vi "swiftCreate.vi"() -> ()   [LabVIEW 2016, in "Cerebellum.lvclass"]
uses:
  Cerebellum.lvclass
  Controls/Type of Synapses.ctl
  Cube/Grid.lvclass
  Cube/Grid.lvclass/Grid.ctl
  AER/AER.lvclass/AER.ctl
  Controls/Type of Neuron.ctl
  <vilib>/Utility/xml.llb/Write to XML File(string).vi
  <vilib>/Utility/file.llb/Write Delimited Spreadsheet.vi
  <vilib>/Utility/file.llb/Write Delimited Spreadsheet (DBL).vi
  <vilib>/Utility/xml.llb/Read From XML File(string).vi
  Synapses/Synapses.lvclass
  AER/AER.lvclass
panel:
  out "Creating grid":dbl(slide) scale=0.0..1.0
  in  "Show":bool
  in  "stop":bool
  in  "Create":bool
  out "Grid":string
  in  "Synapses and parameters":T2(array[cluster])=[{"Conv %"=4.0, "Synapse"=enum."MF to GC", "Weight Gain"=0.4}, {"Conv %"=4.0, "Synapse"=enum."GO to GC", "Weight Gain"=-0.03}, {"Conv %"=0.4, "Synapse"=enum."GC to GO", "Weight Gain"=0.002}, {"Conv %"=0.5, "Synapse"=enum."MF to GO", "Weight Gain"=0.001}, {"Conv %"=0.5, "Synapse"=enum."GC to PC", "Weight Gain"=0.003}, {"Conv %"=0.1, "Synapse"=enum."GC to BA", "Weight Gain"=0.008}, {"Conv %"=0.01, "Synapse"=enum."PC to BA", "Weight Gain"=-0.2}, {"Conv %"=0.4, "Synapse"=enum."BA to PC", "Weight Gain"=-0.01}, {"Conv %"=0.1, "Synapse"=enum."BA to GO", "Weight Gain"=-0.01}]
  in  "Prefix for output files name?":string="aer_"
  in  "How namy maps?":i32=1
  out "Preview":string
  in  "New":bool
  in  "Load":bool
  in  "Existing Grids in Results/":i32(listbox)
  # "Given the Grid, create random synaptic weights, distance based synaptic connections and output AER maps"
  # "Double click on the grid name shows details"
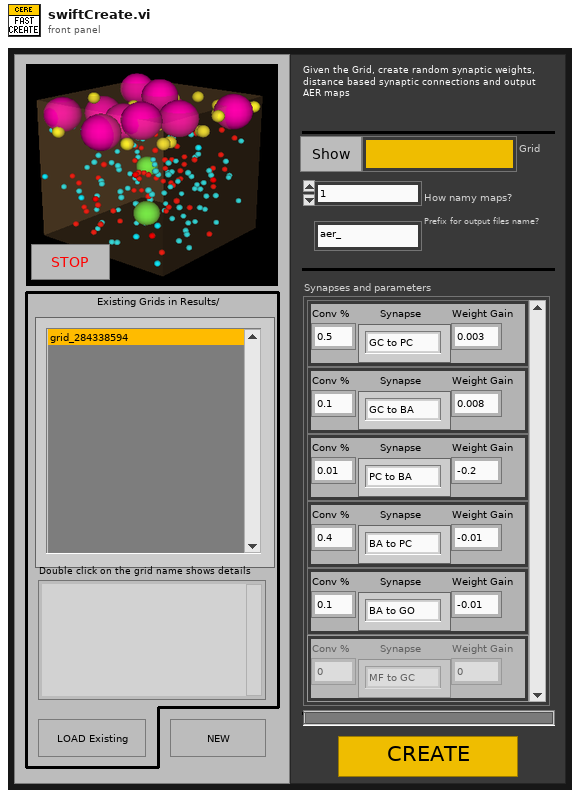
[diagram p1: front panel]
types:
  T1 = typedef "Type of Synapses.ctl" = enum16{"MF to GC", "GO to GC", "GC to GO", "MF to GO", "GC to PC", "GC to BA", "PC to BA", "BA to PC", "BA to GO"}
  T2 = cluster{"Conv %":dbl, "Synapse":T1, "Weight Gain":dbl}[]
  T3 = enum16{"Iddle", "CreateGrid", "CreateMaps", "LoadGrids", "Init", "ShowGrid"}
  T4 = enum8{"Enabled", "Disabled", "Disabled and Grayed Out"}
  T5 = enum16{"Iddle", "CreateGrid", "CreateMaps", "LoadGrids", "Init"}
  T6 = typedef "Type of Neuron.ctl" = enum16{"MF", "BA", "GO", "GC", "PC", "LU", "Glia (Dummy)"}
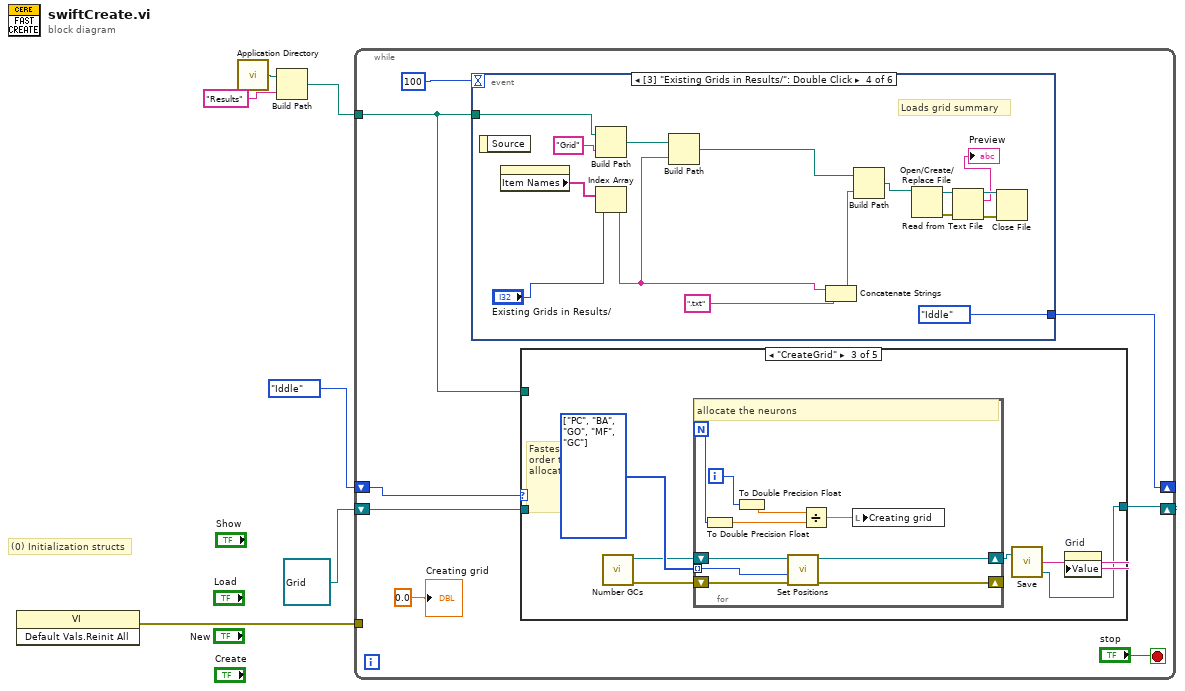
[diagram p0: block diagram]
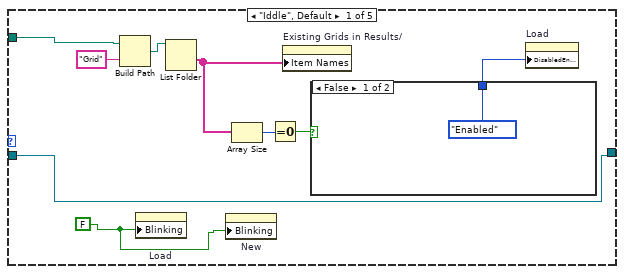
[diagram p2: hidden frame]
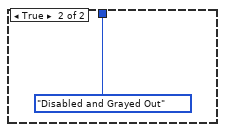
[diagram p3: hidden frame]
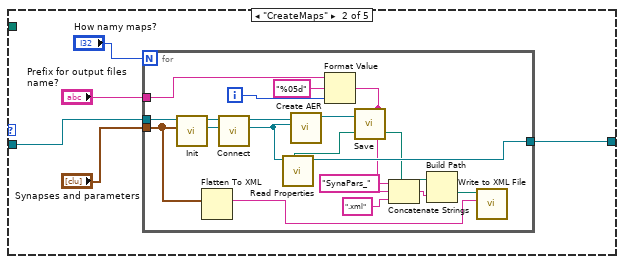
[diagram p4: hidden frame]
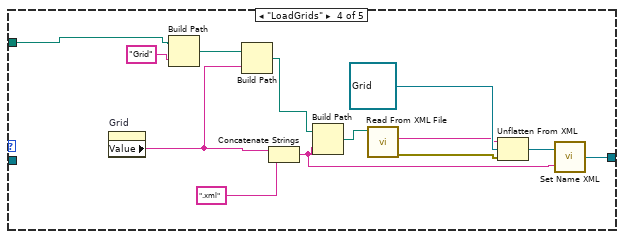
[diagram p5: hidden frame]
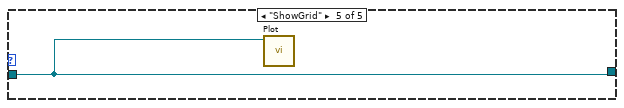
[diagram p6: hidden frame]
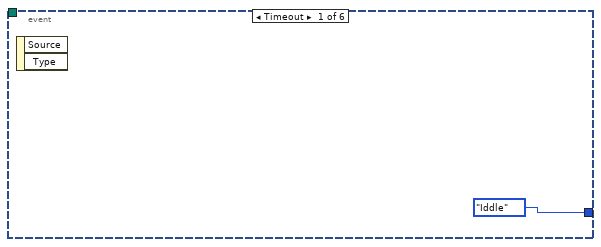
[diagram p7: hidden frame]
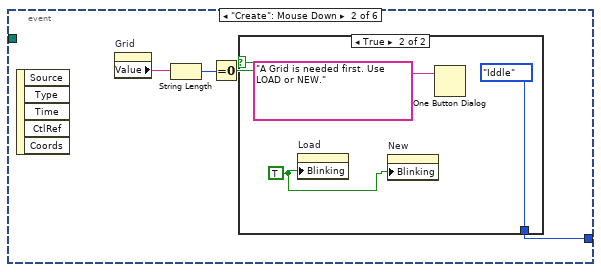
[diagram p8: hidden frame]
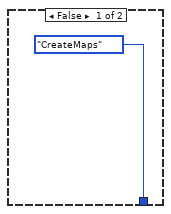
[diagram p9: hidden frame]
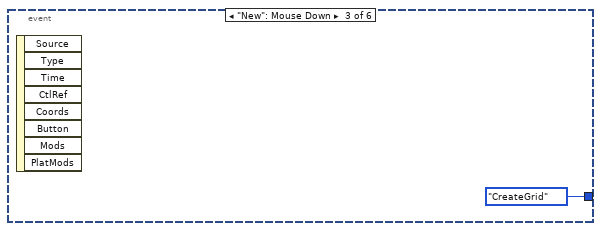
[diagram p10: hidden frame]
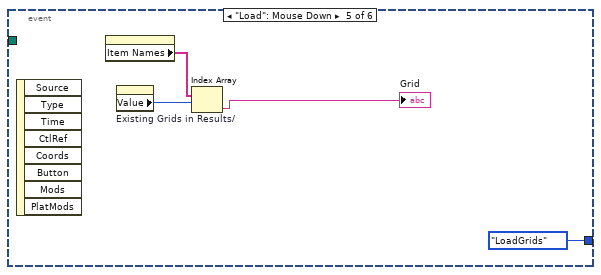
[diagram p11: hidden frame]
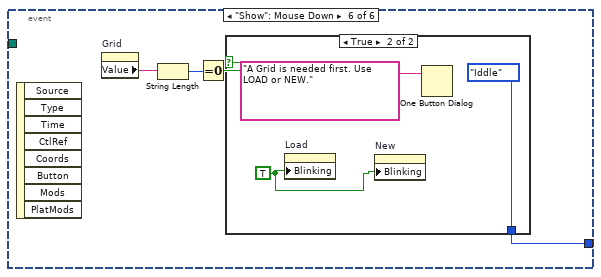
[diagram p12: hidden frame]
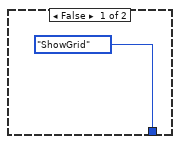
[diagram p13: hidden frame]
diagram:
  # "(0) Initialization structs"
  n1 = invoke class="VI" method="Default Vals.Reinit All"() -> (error out=w1:errorcluster)  [unwired: 3 in, 2 out]
  n2 = call <vilib>:"Application Directory.vi"() -> ("Application Directory"=w6:path)
  n3 = Build Path(base path=w6, name or relative path="Results") -> (appended path=w4:path)
  n4 = while {
    tunnel: w4 -> [w13]
    shift-right: [w12] -> _
    shift-left: T3."Iddle" -> [w8]
    shift-right: [w10] -> _
    shift-left: refnum<class "Grid.lvclass"> refnum ("Cube out") -> [w9]
    tunnel: w1 -> [_]
    stop <- "stop" stop-if-true
    n5 = event shown="[3] \"Existing Grids in Results/\": Double Click" {
      selector: _ -> [_ _ _ _ _ _]
      dyn-events: _ -> [_ _ _ _ _ _]
      timeout: 100 -> [_ _ _ _ _ _]
      tunnel: w13 -> [_ _ _ w94 _ _]
      tunnel: [T3."Iddle" w81 T3."CreateGrid" T5."Iddle" T5."LoadGrids" w110] -> w12
      event Timeout {
        n6 = event-data() -> ()  [unwired: 1 in, 2 out]
      }
      event "Create": Mouse Down {
        n7 = event-data() -> ()  [unwired: 1 in, 5 out]
        n8 = property on="Grid" class="Str"() -> ("Value"=w84:string)  [unwired: 2 in, 2 out]
        n9 = String Length(string=w84) -> (length=w83:i32)
        n10 = Equal To 0?(x=w83) -> (x = 0?=w82:bool)
        n11 = case shown="True" w82 {
          tunnel: [T3."CreateMaps" T3."Iddle"] -> w81
          frame False {
          }
          frame True {
            w86 = TRUE ("Blinking")
            n12 = property on="Load" class="Bool (strict)"("Blinking"=w86) -> ()  [unwired: 2 in, 2 out]
            n13 = property on="New" class="Bool (strict)"("Blinking"=w86) -> ()  [unwired: 2 in, 2 out]
            n14 = One Button Dialog(message="A Grid is needed first. Use LOAD or NEW.") -> ()  [unwired: 1 in, 1 out]
          }
        }
      }
      event "New": Mouse Down {
        n15 = event-data() -> ()  [unwired: 1 in, 8 out]
      }
      event "Existing Grids in Results/": Double Click {
        # "Loads grid summary"
        n16 = event-data() -> ()  [unwired: 1 in, 1 out]
        n17 = property on="Existing Grids in Results/" class="LstBox (strict)"() -> ("Item Names"=w99:string[])  [unwired: 2 in, 2 out]
        n18 = Build Path(base path=w94, name or relative path="Grid") -> (appended path=w91:path)
        n19 = Index Array(array=w99, index="Existing Grids in Results/") -> (element=w90:string)
        n20 = Build Path(base path=w91, name or relative path=w90) -> (appended path=w92:path)
        n21 = Concatenate Strings(w90, ".txt" ("string")) -> (w96:string)
        n22 = Build Path(base path=w92, name or relative path=w96) -> (appended path=w105:path)
        n23 = Open/Create/Replace File(file path (use dialog)=w105) -> (refnum out=w103:refnum<file>, error out=w104:errorcluster)  [unwired: 5 in, 1 out]
        n24 = Read from Text File(file (use dialog)=w103, error in=w104) -> (refnum out=w101:refnum<file>, text=→"Preview":string, error out=w102:errorcluster)  [unwired: 2 in, 1 out]
        n25 = Close File(refnum=w101, error in=w102) -> ()  [unwired: 2 out]
      }
      event "Load": Mouse Down {
        n26 = event-data() -> ()  [unwired: 1 in, 8 out]
        n27 = property on="Existing Grids in Results/" class="LstBox (strict)"() -> ("Item Names"=w108:string[])  [unwired: 2 in, 2 out]
        n28 = property on="Existing Grids in Results/" class="LstBox (strict)"() -> ("Value"=w107:i32)  [unwired: 2 in, 2 out]
        n29 = Index Array(array=w108, index=w107) -> (element=→"Grid":string)
      }
      event "Show": Mouse Down {
        n30 = event-data() -> ()  [unwired: 1 in, 8 out]
        n31 = property on="Grid" class="Str"() -> ("Value"=w113:string)  [unwired: 2 in, 2 out]
        n32 = String Length(string=w113) -> (length=w112:i32)
        n33 = Equal To 0?(x=w112) -> (x = 0?=w111:bool)
        n34 = case shown="True" w111 {
          tunnel: [T3."ShowGrid" T3."Iddle"] -> w110
          frame False {
          }
          frame True {
            w115 = TRUE ("Blinking")
            n35 = property on="Load" class="Bool (strict)"("Blinking"=w115) -> ()  [unwired: 2 in, 2 out]
            n36 = property on="New" class="Bool (strict)"("Blinking"=w115) -> ()  [unwired: 2 in, 2 out]
            n37 = One Button Dialog(message="A Grid is needed first. Use LOAD or NEW.") -> ()  [unwired: 1 in, 1 out]
          }
        }
      }
    }
    n38 = case shown="\"CreateGrid\"" w8 {
      tunnel: w13 -> [w18 _ _ w70 _]
      tunnel: [w16 w26 w51 w66 w79] -> w10
      tunnel: w9 -> [w16 w30 _ _ w79]
      frame "Iddle", Default {
        w15 = FALSE ("Blinking")
        n39 = Build Path(base path=w18, name or relative path="Grid") -> (appended path=w19:path)
        n40 = property on="Load" class="Bool (strict)"("Blinking"=w15) -> ()  [unwired: 2 in, 2 out]
        n41 = List Folder(path=w19) -> (folder names=w17:string[])  [unwired: 3 in, 3 out]
        n42 = property on="New" class="Bool (strict)"("Blinking"=w15) -> ()  [unwired: 2 in, 2 out]
        n43 = Array Size(array=w17) -> (size(s)=w23:i32)
        n44 = Equal To 0?(x=w23) -> (x = 0?=w22:bool)
        n45 = property on="Existing Grids in Results/" class="LstBox (strict)"("Item Names"=w17) -> ()  [unwired: 2 in, 2 out]
        n46 = case shown="False" w22 {
          tunnel: [T4."Enabled" ("Disabled") T4."Disabled and Grayed Out" ("Disabled")] -> w21
          frame False {
          }
          frame True {
          }
        }
        n47 = property on="Load" class="Bool (strict)"("DisabledEnum"=w21) -> ()  [unwired: 2 in, 2 out]
      }
      frame "CreateMaps" {
        n48 = for {
          N: "How namy maps?" -> [_]
          tunnel: w30 -> [w47]
          tunnel: "Synapses and parameters" -> [w34]
          tunnel: "Prefix for output files name?" -> [w42]
          tunnel: [w43] -> w26
          i -> [w40]
          n49 = call "Init.vi"("Info Synapses"=w34, "Grid in"=w47) -> ("Grid out"=w49:refnum<class "Grid.lvclass">, "Synapses out"=w48:refnum<class "Synapses.lvclass">)  [unwired: 8 in]
          n50 = Flatten To XML(anything=w34) -> (xml string=w32:string)
          n51 = call "Connect.vi"("Grid in"=w49, "Synapses in"=w48) -> ("Grid out"=w44:refnum<class "Grid.lvclass">, "Synapses  out"=w45:refnum<class "Synapses.lvclass">)  [unwired: 8 in]
          n52 = call "Read Properties.vi"("Grid in"=w44) -> ("Grid out"=w43:refnum<class "Grid.lvclass">, "Path"=w38:path)  [unwired: 3 in, 6 out]
          n53 = call "Create AER.vi"("Grid.lvclass"=w44, "Synapses in"=w45) -> ("AER.lvclass"=w46:refnum<class "AER.lvclass">)  [unwired: 6 in, 3 out]
          n54 = Format Value(string ("")=w42, format string="%05d", value (0)=w40) -> (output string=w36:string)
          n55 = call "Save.vi"("AER file name"=w36, "Inpath"=w38, "AER in"=w46) -> ("created path"=w31:path)
          n56 = Concatenate Strings("SynaPars_" ("string"), w36, ".xml" ("name or relative path")) -> (w39:string)
          n57 = Build Path(base path=w31, name or relative path=w39) -> (appended path=w35:path)
          n58 = call-poly <vilib>:"Write to XML File.vi"("XML Input"=w32, "XML File Path"=w35) -> ()  [unwired: 7 in, 3 out]
        }
      }
      frame "CreateGrid" {
        w55 = T6[] [enum."PC", enum."BA", enum."GO", enum."MF", enum."GC"] items=["MF", "BA", "GO", "GC", "PC", "LU", "Glia (Dummy)"]
        # "Fastes order to allocate"
        n59 = call "Number GCs.vi"() -> ("error out"=w54:errorcluster, "Cube out"=w50:refnum<class "Grid.lvclass">)  [unwired: 5 in, 2 out]
        n60 = for {
          N -> [w60]
          shift-right: [w64] -> w53
          shift-left: w50 -> [w65]
          tunnel: w55 -> [w61] mode=indexing
          shift-right: [w62] -> _
          shift-left: w54 -> [w63]
          i -> [w57]
          # "allocate the neurons"
          n61 = To Double Precision Float(number=w60) -> (double precision float=w58:dbl)
          n62 = To Double Precision Float(number=w57) -> (double precision float=w59:dbl)
          n63 = call "Set Positions.vi"("error in"=w63, "Type of Neuron"=w61, "Grid in"=w65) -> ("error out"=w62:errorcluster, "Grid out"=w64:refnum<class "Grid.lvclass">)  [unwired: 7 in]
          n64 = Divide(x=w59, y=w58) -> (x/y=w56:dbl)
          n65 = local write "Creating grid"(w56) -> ()
        }
        n66 = call "Save.vi"("Grid in"=w53) -> ("FileName"=w52:string, "Grid out"=w51:refnum<class "Grid.lvclass">)  [unwired: 1 in, 1 out]
        n67 = property on="Grid" class="Str"("Value"=w52) -> ()  [unwired: 2 in, 2 out]
      }
      frame "LoadGrids" {
        n68 = property on="Grid" class="Str"() -> ("Value"=w68:string)  [unwired: 2 in, 2 out]
        n69 = Build Path(base path=w70, name or relative path="Grid") -> (appended path=w72:path)
        n70 = Build Path(base path=w72, name or relative path=w68) -> (appended path=w69:path)
        n71 = Concatenate Strings(w68, ".xml" ("string")) -> (w67:string)
        n72 = Build Path(base path=w69, name or relative path=w67) -> (appended path=w75:path)
        n73 = call-poly <vilib>:"Read From XML File.vi"("XML File Path"=w75) -> ("error out"=w76:errorcluster, "XML Elements"=w74:string)  [unwired: 8 in, 1 out]
        n74 = Unflatten From XML(xml string=w74, type=refnum<class "Grid.lvclass"> refnum ("Grid in"), error in (no error)=w76) -> (value=w78:refnum<class "Grid.lvclass">)  [unwired: 1 out]
        n75 = call-dynamic "Set Name XML.vi"("Name XML File"=w67, "Grid in"=w78) -> ("Grid out"=w66:refnum<class "Grid.lvclass">)
      }
      frame "ShowGrid" {
        n76 = call "Plot.vi"("Grid in"=w79) -> ()  [unwired: 11 in]
      }
    }
    "Creating grid" <- 0.0 ("Creating grid")
  }
